vi "IMAQdx Acquisition Template (Host)forRT.vi"() -> ()   [LabVIEW 2016]
uses:
  <vilib>/rvi/interface/nirviOpenFPGA/nirviOpenFPGA.xnode
  <vilib>/rvi/interface/nirviCloseFPGA/nirviCloseFPGA.xnode
  <vilib>/rvi/interface/nirviMethod/nirviMethod.xnode
  <vilib>/FPGAPlugInAG/Dynamic/niLvFpga_Close_Dynamic.vi
  <vilib>/vision/driver/NI_Vision_Acquisition_Software.lvlib
  <resource>/objmgr/imaqdx.rc
  <vilib>/vision/driver/IMAQdx.llb/IMAQdx Acquisition Mode.ctl
  <vilib>/vision/driver/IMAQdx.llb/IMAQdx Buffer Number Mode.ctl
  <vilib>/visionFPGA/NI_VDM_FPGA_Basics.lvlib
  <vilib>/FPGAPlugInAG/Dynamic/niLvFpga_Download_Dynamic.vi
  <vilib>/FPGAPlugInAG/Dynamic/niLvFpga_Run_Dynamic.vi
  <vilib>/rvi/interface/nirviReadWriteControl/nirviReadWriteControl.xnode
  <vilib>/rvi/interface/Simulation/niFpgaSimulationCallBeginRW.vi
  <vilib>/rvi/errors/niLvFpgaAdjustHostInterfaceError.vi
  <vilib>/rvi/errors/niLvFpgaMergeErrorWithErrorCode.vi
  <vilib>/FPGAPlugInAG/Dynamic/niLvFpga_ReadFifo_Dynamic.vi
  <vilib>/FPGAPlugInAG/Dynamic/niLvFpga_ConfigureFifo_Dynamic.vi
  <vilib>/FPGAPlugInAG/Dynamic/niLvFpga_StartFifo_Dynamic.vi
  <vilib>/visionFPGA/Basics/Image Transfer to Target/IMAQ FPGA Image Transfer to Target U32.vi
  <vilib>/visionFPGA/Basics/Configure Image Transfer to Target/IMAQ FPGA Configure Image Transfer to Target U32.vi
  <vilib>/userdefined/High Color/IMAQdx.ctl
  FPGA Bitfiles/ImageProcessingw_FPGATarget2_ImageProcessingw_ZcF2hsHpmf8.lvbitx
  <vilib>/FPGAPlugInAG/roboRIO/niLvFpga_Open_roboRIO.vi
  <vilib>/rvi/interface/common/dynamic/niFpgaDynamicAddResources.vi
panel:
  out "error out":errorcluster
  out "dePixelCount":u32
  out "AllPixelCount":u32
  out "OriImage Err out":errorcluster
  out "Image":T1(plugin-control)
  out "error out 2":errorcluster
  out "Error Out":errorcluster
  in  "Stop":bool
  # "Overview: Demonstrates how to acquire an image from a camera using the IMAQdx API, transfer the image to a FPGA target for processing, and retrieve the processed image for display or further processing on the host.\nRequirements:\n- LabVIEW FPGA\n- Vision Acquisition Software\n- Vision Development Module\nInstructions:\n1. Select a Camera\n2. Run the VI."
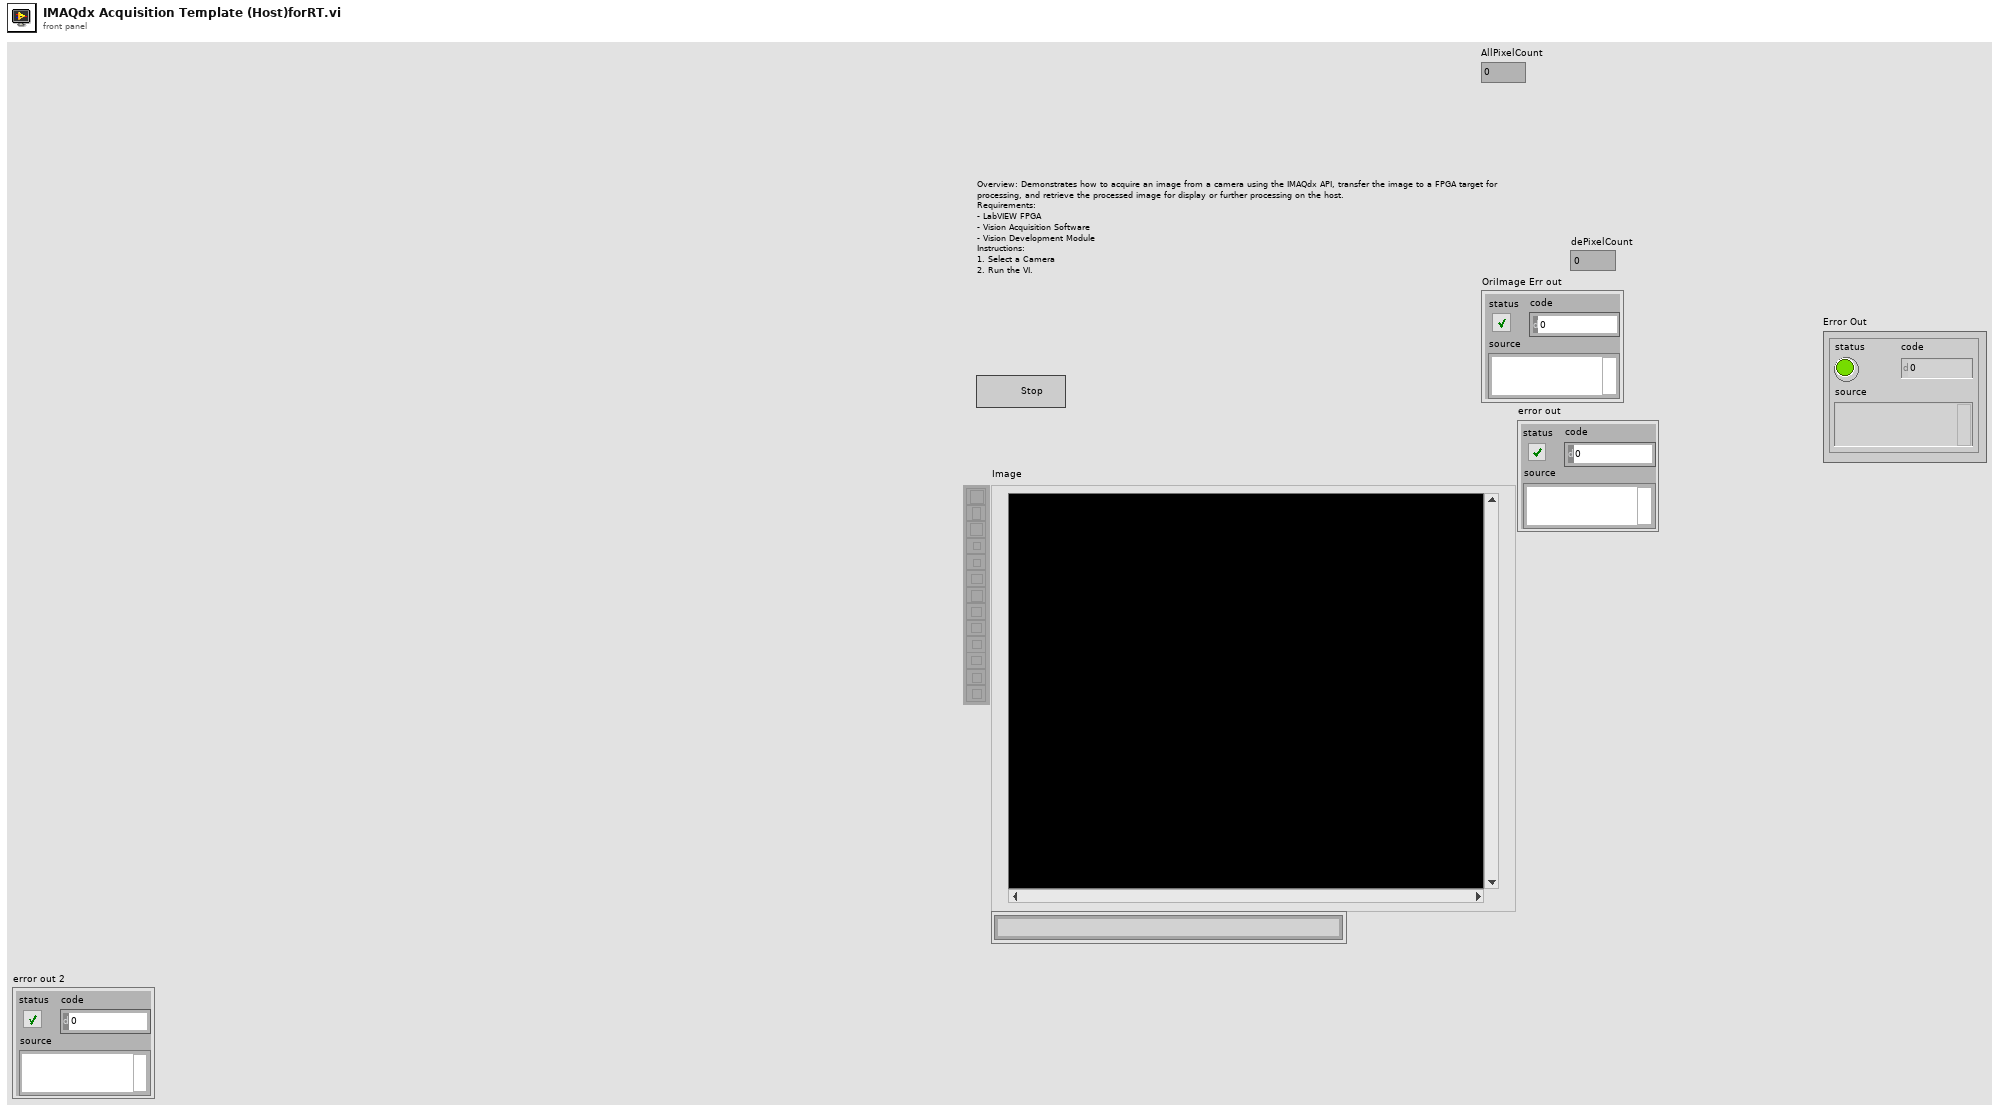
[diagram p1: front panel]
types:
  T1 = typedef "IMAQ Image.ctl" = refnum<image>
  T2 = typedef "IMAQdx.ctl" = refnum<k21>
  T3 = typedef "Image Type" = u32
  T4 = typedef "NI_Vision_Acquisition_Software.lvlib/IMAQdx Acquisition Mode.ctl" = enum32{"One Shot", "Continuous"}
  T5 = typedef "NI_Vision_Acquisition_Software.lvlib/IMAQdx Buffer Number Mode.ctl" = enum32{"Next", "Last", "Buffer Number", "Every", "Last New"}
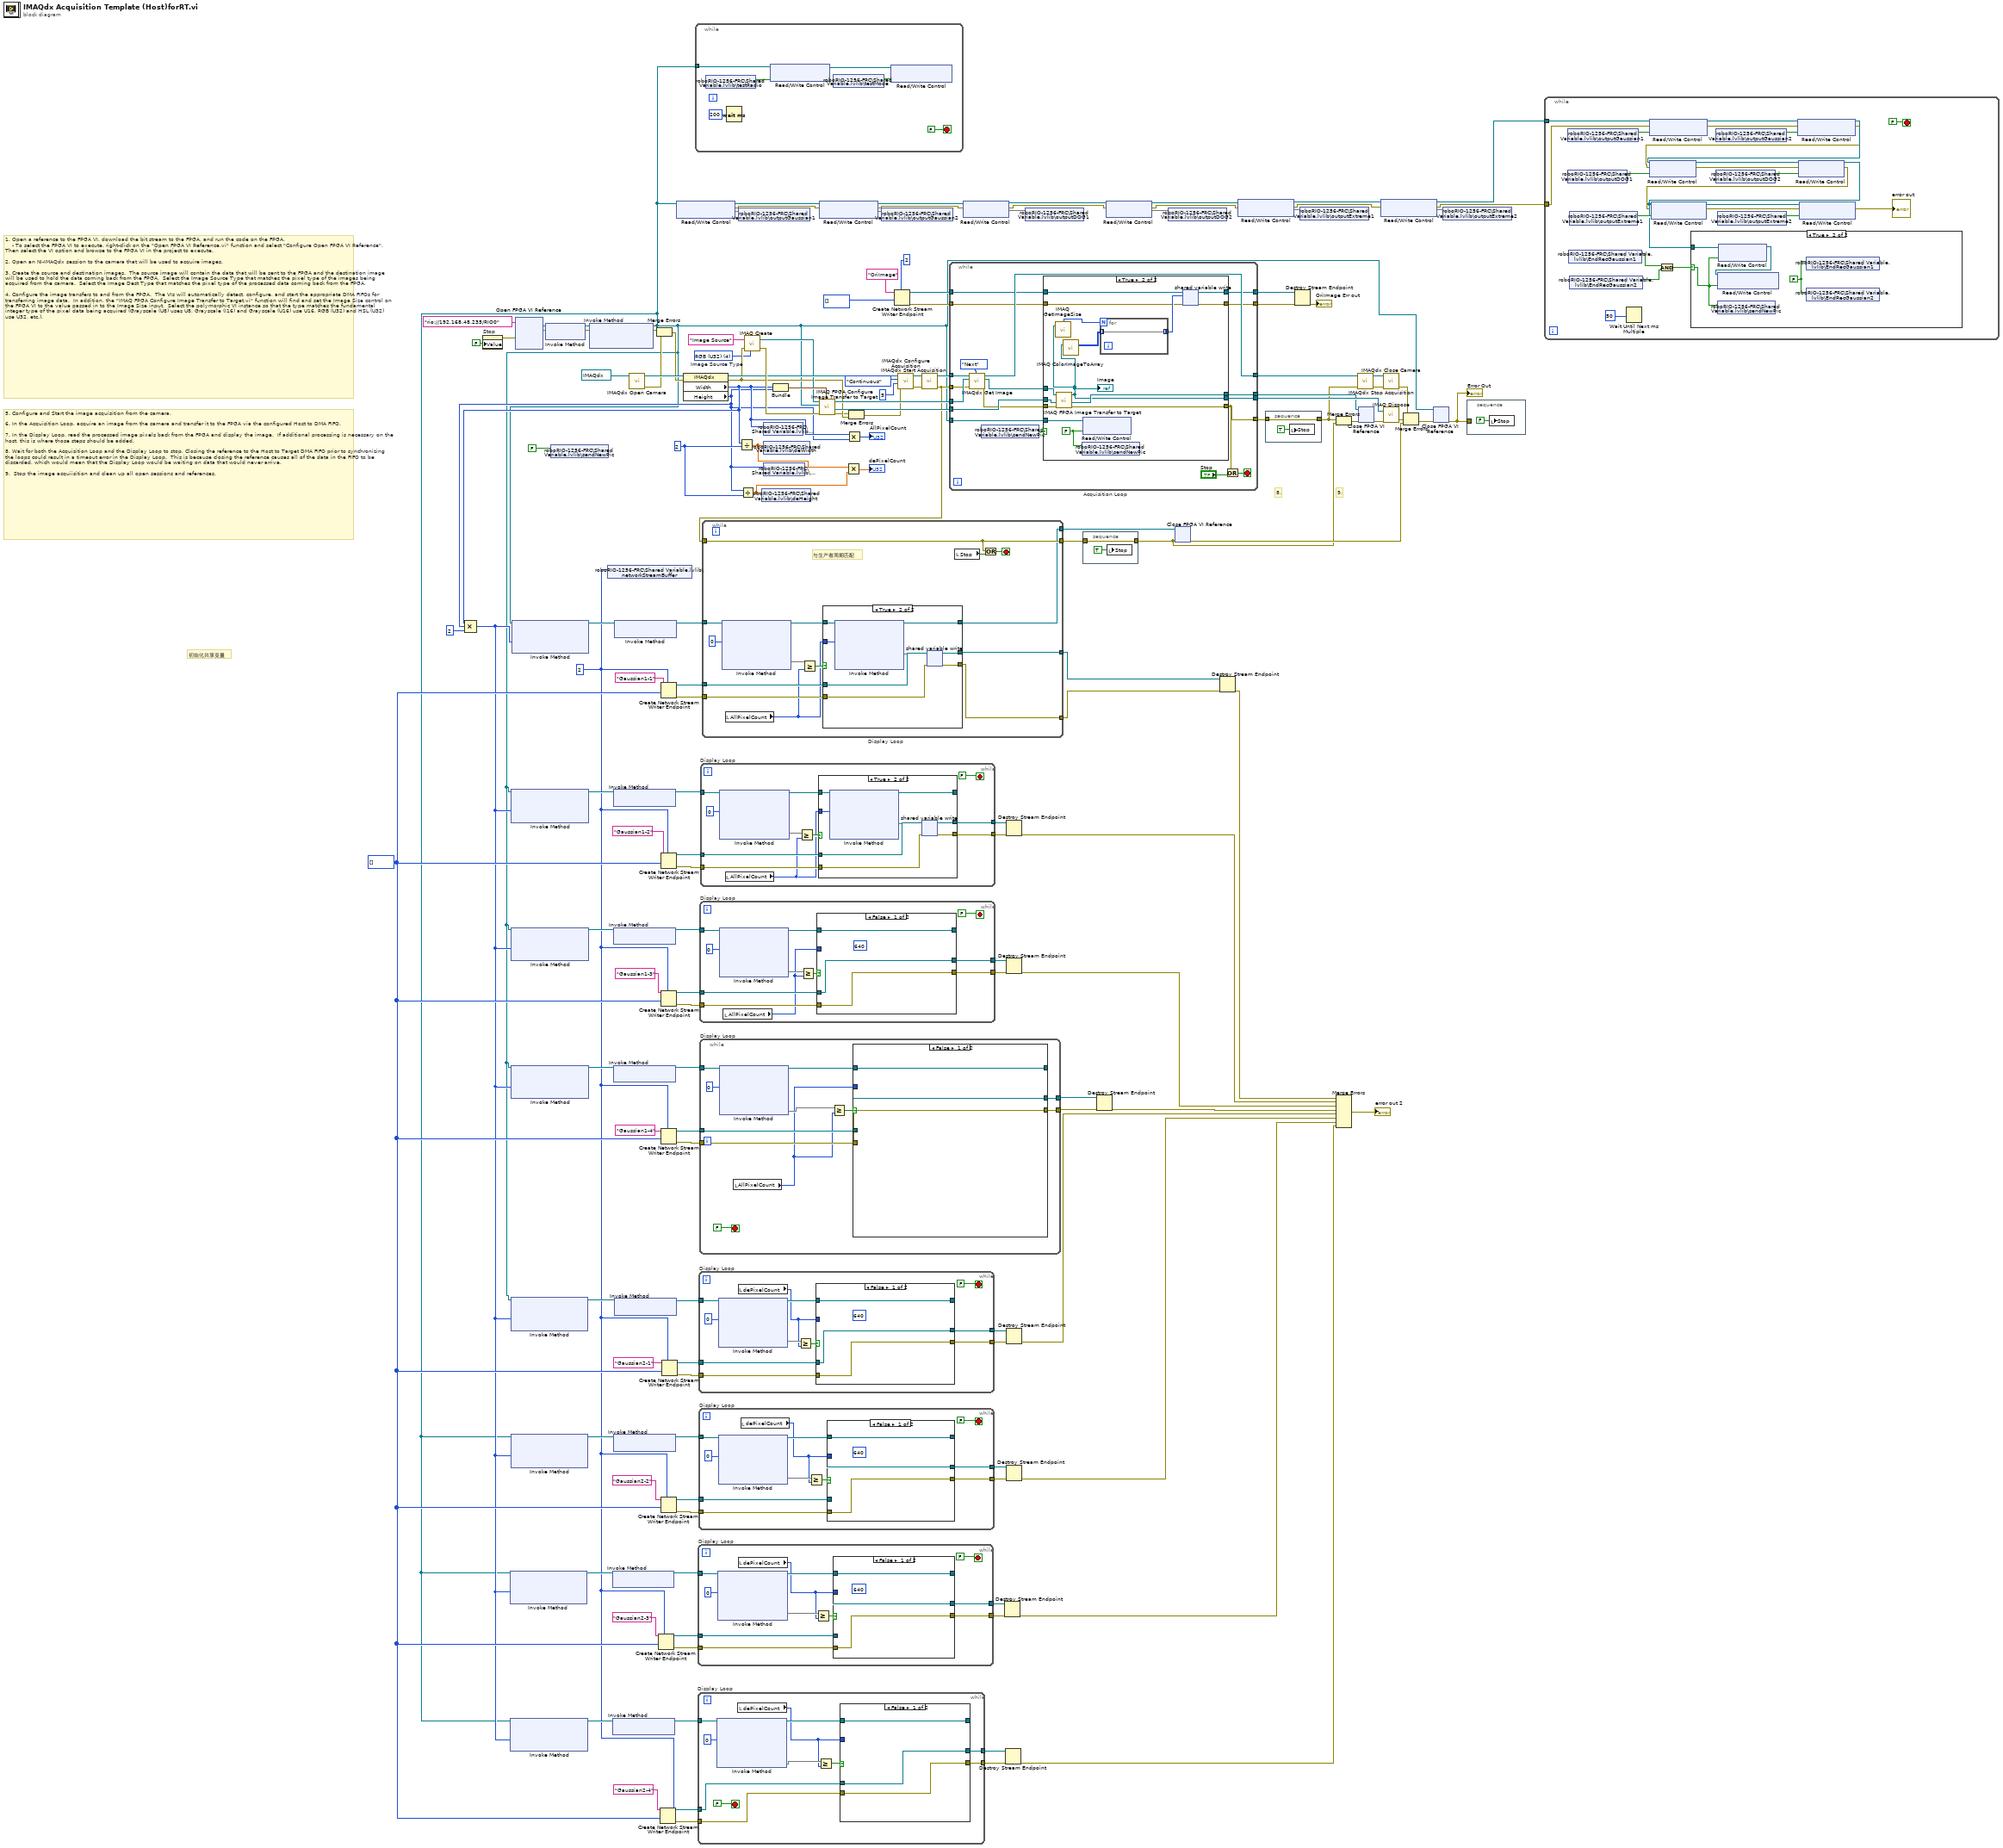
[diagram p0: block diagram]
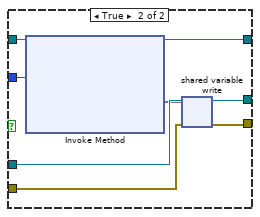
[diagram p3: hidden frame]
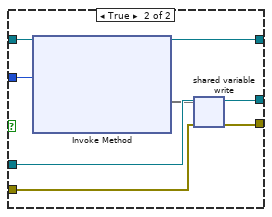
[diagram p4: hidden frame]
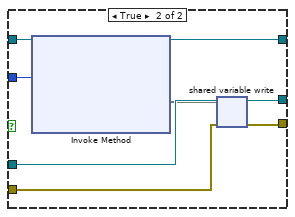
[diagram p5: hidden frame]
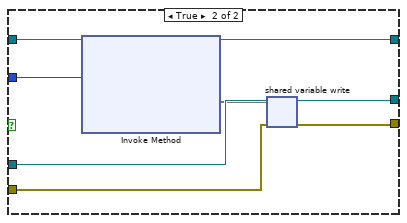
[diagram p6: hidden frame]
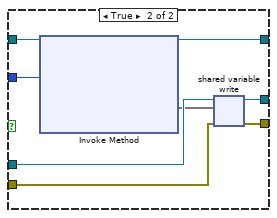
[diagram p7: hidden frame]
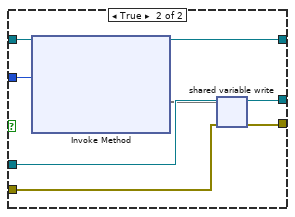
[diagram p8: hidden frame]
diagram:
  w27 = u32 2 ("y")
  w37 = i32[] []
  w34 = 2 ("writer buffer size")
  w114 = T3 4 items=["Grayscale (U8)", "Grayscale (I16)", "Grayscale (SGL)", "Complex (CSG)", "RGB (U32)", "HSL (U32)", "RGB (U64)", "Grayscale (U16)"]  # Image Source Type
  # "初始化共享变量"
  # "5. Configure and Start the image acquisition from the camera.\n\n6. In the Acquisition Loop, acquire an image from the camera and transfer it to the FPGA via the configured Host to DMA FIFO.\n\n7. In the Display Loop, read the processed image pixels back from the FPGA and display the image.  If additional processing is necessary on the host, this is where those steps should be added.\n\n8. Wait for both the Acquisition Loop and the Display Loop to stop. Closing the reference to the Host to Target DMA FIFO prior to synchronizing the loops could result in a timeout error in the Display Loop.  This is because closing the reference causes all of the data in the FIFO to be discarded, which would mean that the Display Loop would be waiting on data that would never arrive.\n\n9.  Stop the image acquiisition and clean up all open sessions and references."
  # "1. Open a reference to the FPGA VI, download the bit stream to the FPGA, and run the code on the FPGA.\n    - To select the FPGA VI to execute, right-click on the \"Open FPGA VI Reference.vi\" function and select \"Configure Open FPGA VI Reference\".  Then select the VI option and browse to the FPGA VI in the project to execute.\n\n2. Open an NI-IMAQdx session to the camera that will be used to acquire images.\n\n3. Create the source and destination images.  The source image will contain the data that will be sent to the FPGA and the destination image will be used to hold the data coming back from the FPGA.  Select the Image Source Type that matches the pixel type of the images being acquired from the camera.  Select the Image Dest Type that matches the pixel type of the processed data coming back from the FPGA.\n\n4. Configure the image transfers to and from the FPGA.  The VIs will automatically detect, configure, and start the appropriate DMA FIFOs for transferring image data.  In addition, the \"IMAQ FPGA Configure Image Transfer to Target.vi\" function will find and set the Image Size control on the FPGA VI to the value passed in to the Image Size input.  Select the polymorphic VI instance so that the type matches the fundamental integer type of the pixel data being acquired (Grayscale (U8) uses U8, Grayscale (I16) and Grayscale (U16) use U16, RGB (U32) and HSL (U32) use U32, etc.)."
  # "9."
  # "8."
  n1 = property on="Stop" class="Bool (strict)"("Value"=FALSE ("Stop")) -> (error out=w149:errorcluster)  [unwired: 2 in, 1 out]
  n2 = xnode "Open FPGA VI Reference"("error in"=w149, "resource name"=tag "rio://192.168.48.235/RIO0") -> ("FPGA VI Reference Out"=w145:refnum<k20>, "error out"=w146:errorcluster)
  n3 = xnode "Invoke Method"("FPGA VI Reference In"=w145, "error in"=w146) -> ("FPGA VI Reference Out"=w148:refnum<k20>, "error out"=w147:errorcluster)
  n4 = shared-variable "roboRIO-1256-FRC\\Shared Variable.lvlib\\sendNewPic"(FALSE) -> ()  [unwired: 1 in, 1 out]
  n5 = xnode "Invoke Method"("FPGA VI Reference In"=w148, "error in"=w147) -> ("FPGA VI Reference Out"=w1:refnum<k20>, "error out"=w134:errorcluster)  [unwired: 1 in]
  n6 = shared-variable "roboRIO-1256-FRC\\Shared Variable.lvlib\\networkStreamBuffer"(w34) -> ()  [unwired: 1 in, 1 out]
  n7 = call <vilib>:"IMAQdx Open Camera.vi"("Session In"=T2 "cam0" ("Camera")) -> ("error out"=w119:errorcluster, "Session Out"=w120:T2)  [unwired: 9 in]
  n8 = Merge Errors(w134, w119) -> (w118:errorcluster)
  n9 = Create Network Stream Writer Endpoint(7:w34, 9:w37, 11:"Gaussian2-3" ("writer name")) -> (0:w41:errorcluster, 3:w40:refnum<k21>)  [unwired: 4 in]
  n10 = Create Network Stream Writer Endpoint(7:w34, 9:w37, 11:"Gaussian2-4" ("writer name")) -> (0:w66:errorcluster, 3:w67:refnum<k21>)  [unwired: 4 in]
  n11 = Create Network Stream Writer Endpoint(7:w34, 9:w37, 11:"Gaussian2-2" ("writer name")) -> (0:w48:errorcluster, 3:w49:refnum<k21>)  [unwired: 4 in]
  n12 = Create Network Stream Writer Endpoint(7:w34, 9:w37, 11:"Gaussian1-1" ("writer name")) -> (0:w98:errorcluster, 3:w97:refnum<k21>)  [unwired: 4 in]
  n13 = Create Network Stream Writer Endpoint(7:w34, 9:w37, 11:"Gaussian1-2" ("writer name")) -> (0:w81:errorcluster, 3:w82:refnum<k21>)  [unwired: 4 in]
  n14 = Create Network Stream Writer Endpoint(7:w34, 9:w37, 11:"Gaussian1-3" ("writer name")) -> (0:w76:errorcluster, 3:w75:refnum<k21>)  [unwired: 4 in]
  n15 = Create Network Stream Writer Endpoint(7:w34, 9:w37, 11:"Gaussian1-4" ("writer name")) -> (0:w60:errorcluster, 3:w61:refnum<k21>)  [unwired: 4 in]
  n16 = Create Network Stream Writer Endpoint(7:w34, 9:w37, 11:"Gaussian2-1" ("writer name")) -> (0:w55:errorcluster, 3:w54:refnum<k21>)  [unwired: 4 in]
  n17 = xnode "Read/Write Control"("FPGA VI Reference In"=w1) -> ("FPGA VI Reference Out"=w24:refnum<k20>, "error out"=w8:errorcluster, "outputGaussian1"=w26)  [unwired: 1 in]
  n18 = property class="IMAQdx"(reference=w120, error in=w118) -> (reference out=w127:T2, error out=w115:errorcluster, "Width"=w14:u32, "Height"=w13:u32)
  n19 = Compound Arithmetic op=MULTIPLY(w14, w13, u32 2 ("value")) -> (w33:u32)
  n20 = xnode "Invoke Method"("FPGA VI Reference In"=w1, "Requested Depth"=w33) -> ("FPGA VI Reference Out"=w42:refnum<k20>)  [unwired: 1 in, 2 out]
  n21 = xnode "Invoke Method"("FPGA VI Reference In"=w1, "Requested Depth"=w33) -> ("FPGA VI Reference Out"=w65:refnum<k20>)  [unwired: 1 in, 2 out]
  n22 = xnode "Invoke Method"("FPGA VI Reference In"=w1, "Requested Depth"=w33) -> ("FPGA VI Reference Out"=w36:refnum<k20>)  [unwired: 1 in, 2 out]
  n23 = xnode "Invoke Method"("FPGA VI Reference In"=w1, "Requested Depth"=w33) -> ("FPGA VI Reference Out"=w47:refnum<k20>)  [unwired: 1 in, 2 out]
  n24 = xnode "Invoke Method"("FPGA VI Reference In"=w1, "Requested Depth"=w33) -> ("FPGA VI Reference Out"=w80:refnum<k20>)  [unwired: 1 in, 2 out]
  n25 = xnode "Invoke Method"("FPGA VI Reference In"=w1, "Requested Depth"=w33) -> ("FPGA VI Reference Out"=w77:refnum<k20>)  [unwired: 1 in, 2 out]
  n26 = xnode "Invoke Method"("FPGA VI Reference In"=w1, "Requested Depth"=w33) -> ("FPGA VI Reference Out"=w59:refnum<k20>)  [unwired: 1 in, 2 out]
  n27 = xnode "Invoke Method"("FPGA VI Reference In"=w1, "Requested Depth"=w33) -> ("FPGA VI Reference Out"=w104:refnum<k20>)  [unwired: 1 in, 2 out]
  n28 = xnode "Invoke Method"("FPGA VI Reference In"=w42) -> ("FPGA VI Reference Out"=w43:refnum<k20>)  [unwired: 1 in, 1 out]
  n29 = xnode "Invoke Method"("FPGA VI Reference In"=w65) -> ("FPGA VI Reference Out"=w64:refnum<k20>)  [unwired: 1 in, 1 out]
  n30 = xnode "Invoke Method"("FPGA VI Reference In"=w47) -> ("FPGA VI Reference Out"=w46:refnum<k20>)  [unwired: 1 in, 1 out]
  n31 = xnode "Invoke Method"("FPGA VI Reference In"=w80) -> ("FPGA VI Reference Out"=w79:refnum<k20>)  [unwired: 1 in, 1 out]
  n32 = xnode "Invoke Method"("FPGA VI Reference In"=w77) -> ("FPGA VI Reference Out"=w78:refnum<k20>)  [unwired: 1 in, 1 out]
  n33 = xnode "Invoke Method"("FPGA VI Reference In"=w59) -> ("FPGA VI Reference Out"=w58:refnum<k20>)  [unwired: 1 in, 1 out]
  n34 = xnode "Invoke Method"("FPGA VI Reference In"=w104) -> ("FPGA VI Reference Out"=w103:refnum<k20>)  [unwired: 1 in, 1 out]
  n35 = xnode "Invoke Method"("FPGA VI Reference In"=w36) -> ("FPGA VI Reference Out"=w35:refnum<k20>)  [unwired: 1 in, 1 out]
  n36 = while {
    tunnel: w1 -> [w151]
    stop <- FALSE stop-if-true
    n37 = shared-variable "roboRIO-1256-FRC\\Shared Variable.lvlib\\testRadio"() -> (w152:bool)  [unwired: 1 in, 1 out]
    n38 = Wait (ms)(milliseconds to wait=u32 200) -> ()  [unwired: 1 out]
    n39 = xnode "Read/Write Control"("FPGA VI Reference In"=w151, "Radio LED Status"=w152) -> ("FPGA VI Reference Out"=w156:refnum<k20>)  [unwired: 1 in, 1 out]
    n40 = shared-variable "roboRIO-1256-FRC\\Shared Variable.lvlib\\testMode"() -> (w153:bool)  [unwired: 1 in, 1 out]
    n41 = xnode "Read/Write Control"("FPGA VI Reference In"=w156, "Comm LED Status"=w153) -> ()  [unwired: 1 in, 2 out]
  }
  n42 = while "Display Loop" {
    tunnel: [w167] -> w70
    tunnel: w66 -> [w166]
    tunnel: w67 -> [w165]
    tunnel: [w161] -> w69
    tunnel: w64 -> [w160]
    stop <- FALSE stop-if-true
    n43 = xnode "Invoke Method"("FPGA VI Reference In"=w160, "Number of Elements"=u32 0) -> ("FPGA VI Reference Out"=w163:refnum<k20>, "Elements Remaining"=w158)  [unwired: 2 in, 2 out]
    n44 = local read "dePixelCount"() -> (w157:u32)
    n45 = Greater Or Equal?(x=w158, y=w157) -> (x >= y?=w159:bool)
    n46 = case shown="False" w159 {
      tunnel: w163 -> [w168 w178]
      tunnel: [w170 w177] -> w167
      tunnel: w166 -> [w169 w176]
      tunnel: w165 -> [w170 w175]
      tunnel: [w169 w174] -> w161
      tunnel: [w168 w173] -> _
      tunnel: w157 -> [_ w171]
      frame False {
      }
      frame True {
        n47 = xnode "Invoke Method"("FPGA VI Reference In"=w178, "Number of Elements"=w171) -> ("FPGA VI Reference Out"=w173:refnum<k20>, "Data"=w172:void[])  [unwired: 2 in, 2 out]
        n48 = shared-variable-write(w175, w176, w172) -> (w177:refnum<k21>, w174:errorcluster)  [unwired: 1 in, 1 out]
      }
    }
  }
  n49 = while "Display Loop" {
    tunnel: [w189] -> w38
    tunnel: w41 -> [w188]
    tunnel: w40 -> [w187]
    tunnel: [w183] -> w39
    tunnel: w43 -> [w182]
    stop <- FALSE stop-if-true
    (unwired) u32 640 ("Number of Elements")
    n50 = xnode "Invoke Method"("FPGA VI Reference In"=w182, "Number of Elements"=u32 0) -> ("FPGA VI Reference Out"=w185:refnum<k20>, "Elements Remaining"=w180)  [unwired: 2 in, 2 out]
    n51 = local read "dePixelCount"() -> (w179:u32)
    n52 = Greater Or Equal?(x=w180, y=w179) -> (x >= y?=w181:bool)
    n53 = case shown="False" w181 {
      tunnel: w185 -> [w190 w200]
      tunnel: [w192 w199] -> w189
      tunnel: w188 -> [w191 w198]
      tunnel: w187 -> [w192 w197]
      tunnel: [w191 w196] -> w183
      tunnel: [w190 w194] -> _
      tunnel: w179 -> [_ w193]
      frame False {
      }
      frame True {
        n54 = xnode "Invoke Method"("FPGA VI Reference In"=w200, "Number of Elements"=w193) -> ("FPGA VI Reference Out"=w194:refnum<k20>, "Data"=w195:void[])  [unwired: 2 in, 2 out]
        n55 = shared-variable-write(w197, w198, w195) -> (w199:refnum<k21>, w196:errorcluster)  [unwired: 1 in, 1 out]
      }
    }
  }
  n56 = while "Display Loop" {
    tunnel: [w211] -> w52
    tunnel: w55 -> [w210]
    tunnel: w54 -> [w209]
    tunnel: [w205] -> w53
    tunnel: w35 -> [w204]
    stop <- FALSE stop-if-true
    (unwired) u32 640 ("Number of Elements")
    n57 = xnode "Invoke Method"("FPGA VI Reference In"=w204, "Number of Elements"=u32 0) -> ("FPGA VI Reference Out"=w207:refnum<k20>, "Elements Remaining"=w202)  [unwired: 2 in, 2 out]
    n58 = local read "dePixelCount"() -> (w201:u32)
    n59 = Greater Or Equal?(x=w202, y=w201) -> (x >= y?=w203:bool)
    n60 = case shown="False" w203 {
      tunnel: w207 -> [w212 w222]
      tunnel: [w214 w221] -> w211
      tunnel: w210 -> [w213 w220]
      tunnel: w209 -> [w214 w219]
      tunnel: [w213 w218] -> w205
      tunnel: [w212 w216] -> _
      tunnel: w201 -> [_ w215]
      frame False {
      }
      frame True {
        n61 = xnode "Invoke Method"("FPGA VI Reference In"=w222, "Number of Elements"=w215) -> ("FPGA VI Reference Out"=w216:refnum<k20>, "Data"=w217:void[])  [unwired: 2 in, 2 out]
        n62 = shared-variable-write(w219, w220, w217) -> (w221:refnum<k21>, w218:errorcluster)  [unwired: 1 in, 1 out]
      }
    }
  }
  n63 = while "Display Loop" {
    tunnel: [w233] -> w51
    tunnel: w48 -> [w232]
    tunnel: w49 -> [w231]
    tunnel: [w227] -> w50
    tunnel: w46 -> [w226]
    stop <- FALSE stop-if-true
    (unwired) u32 640 ("Number of Elements")
    n64 = xnode "Invoke Method"("FPGA VI Reference In"=w226, "Number of Elements"=u32 0) -> ("FPGA VI Reference Out"=w229:refnum<k20>, "Elements Remaining"=w224)  [unwired: 2 in, 2 out]
    n65 = local read "dePixelCount"() -> (w223:u32)
    n66 = Greater Or Equal?(x=w224, y=w223) -> (x >= y?=w225:bool)
    n67 = case shown="False" w225 {
      tunnel: w229 -> [w234 w244]
      tunnel: [w236 w243] -> w233
      tunnel: w232 -> [w235 w242]
      tunnel: w231 -> [w236 w241]
      tunnel: [w235 w240] -> w227
      tunnel: [w234 w238] -> _
      tunnel: w223 -> [_ w237]
      frame False {
      }
      frame True {
        n68 = xnode "Invoke Method"("FPGA VI Reference In"=w244, "Number of Elements"=w237) -> ("FPGA VI Reference Out"=w238:refnum<k20>, "Data"=w239:void[])  [unwired: 2 in, 2 out]
        n69 = shared-variable-write(w241, w242, w239) -> (w243:refnum<k21>, w240:errorcluster)  [unwired: 1 in, 1 out]
      }
    }
  }
  n70 = while "Display Loop" {
    tunnel: [w255] -> w72
    tunnel: w76 -> [w254]
    tunnel: w75 -> [w253]
    tunnel: [w249] -> w73
    tunnel: w78 -> [w248]
    stop <- FALSE stop-if-true
    (unwired) u32 640 ("Number of Elements")
    n71 = xnode "Invoke Method"("FPGA VI Reference In"=w248, "Number of Elements"=u32 0) -> ("FPGA VI Reference Out"=w251:refnum<k20>, "Elements Remaining"=w246)  [unwired: 2 in, 2 out]
    n72 = local read "AllPixelCount"() -> (w245:u32)
    n73 = Greater Or Equal?(x=w246, y=w245) -> (x >= y?=w247:bool)
    n74 = case shown="False" w247 {
      tunnel: w251 -> [w256 w266]
      tunnel: [w258 w265] -> w255
      tunnel: w254 -> [w257 w264]
      tunnel: w253 -> [w258 w263]
      tunnel: [w257 w262] -> w249
      tunnel: [w256 w260] -> _
      tunnel: w245 -> [_ w259]
      frame False {
      }
      frame True {
        n75 = xnode "Invoke Method"("FPGA VI Reference In"=w266, "Number of Elements"=w259) -> ("FPGA VI Reference Out"=w260:refnum<k20>, "Data"=w261:void[])  [unwired: 2 in, 2 out]
        n76 = shared-variable-write(w263, w264, w261) -> (w265:refnum<k21>, w262:errorcluster)  [unwired: 1 in, 1 out]
      }
    }
  }
  n77 = while "Display Loop" {
    tunnel: [w277] -> w63
    tunnel: w60 -> [w276]
    tunnel: w61 -> [w275]
    tunnel: [w271] -> w62
    tunnel: w58 -> [w270]
    stop <- FALSE stop-if-true
    n78 = xnode "Invoke Method"("FPGA VI Reference In"=w270, "Number of Elements"=u32 0) -> ("FPGA VI Reference Out"=w273:refnum<k20>, "Elements Remaining"=w268)  [unwired: 2 in, 2 out]
    n79 = local read "AllPixelCount"() -> (w267:u32)
    n80 = Greater Or Equal?(x=w268, y=w267) -> (x >= y?=w269:bool)
    n81 = case shown="False" w269 {
      tunnel: w273 -> [w278 w282]
      tunnel: [w280 w288] -> w277
      tunnel: w276 -> [w279 w287]
      tunnel: w275 -> [w280 w286]
      tunnel: [w279 w285] -> w271
      tunnel: [w278 w284] -> _
      tunnel: w267 -> [_ w281]
      frame False {
      }
      frame True {
        n82 = xnode "Invoke Method"("FPGA VI Reference In"=w282, "Number of Elements"=w281) -> ("FPGA VI Reference Out"=w284:refnum<k20>, "Data"=w283:void[])  [unwired: 2 in, 2 out]
        n83 = shared-variable-write(w286, w287, w283) -> (w288:refnum<k21>, w285:errorcluster)  [unwired: 1 in, 1 out]
      }
    }
  }
  n84 = while "Display Loop" {
    tunnel: [w299] -> w88
    tunnel: w81 -> [w298]
    tunnel: w82 -> [w297]
    tunnel: [w293] -> w87
    tunnel: w79 -> [w292]
    stop <- FALSE stop-if-true
    (unwired) u32 640 ("Number of Elements")
    n85 = xnode "Invoke Method"("FPGA VI Reference In"=w292, "Number of Elements"=u32 0) -> ("FPGA VI Reference Out"=w295:refnum<k20>, "Elements Remaining"=w290)  [unwired: 2 in, 2 out]
    n86 = local read "AllPixelCount"() -> (w289:u32)
    n87 = Greater Or Equal?(x=w290, y=w289) -> (x >= y?=w291:bool)
    n88 = case shown="True" w291 {
      tunnel: w295 -> [w300 w310]
      tunnel: [w302 w309] -> w299
      tunnel: w298 -> [w301 w308]
      tunnel: w297 -> [w302 w307]
      tunnel: [w301 w306] -> w293
      tunnel: [w300 w304] -> _
      tunnel: w289 -> [_ w303]
      frame False {
      }
      frame True {
        n89 = xnode "Invoke Method"("FPGA VI Reference In"=w310, "Number of Elements"=w303) -> ("FPGA VI Reference Out"=w304:refnum<k20>, "Data"=w305:void[])  [unwired: 2 in, 2 out]
        n90 = shared-variable-write(w307, w308, w305) -> (w309:refnum<k21>, w306:errorcluster)  [unwired: 1 in, 1 out]
      }
    }
  }
  n91 = shared-variable "roboRIO-1256-FRC\\Shared Variable.lvlib\\outputGaussian1"(w26) -> ()  [unwired: 1 in, 1 out]
  n92 = Divide(x=w14, y=w27) -> (x/y=w10:dbl)
  n93 = Divide(x=w13, y=w27) -> (x/y=w9:dbl)
  n94 = call "IMAQ Create"("Image Name"="Image Source", "Image Type"=w114, "error in (no error)"=w115) -> ("New Image"=w125:T1, "error out"=w133:errorcluster)  [unwired: 2 in]
  n95 = shared-variable "roboRIO-1256-FRC\\Shared Variable.lvlib\\deHeight"(w9) -> ()  [unwired: 1 in, 1 out]
  n96 = shared-variable "roboRIO-1256-FRC\\Shared Variable.lvlib\\Width"(w14) -> ()  [unwired: 1 in, 1 out]
  n97 = shared-variable "roboRIO-1256-FRC\\Shared Variable.lvlib\\deWidth"(w10) -> ()  [unwired: 1 in, 1 out]
  n98 = shared-variable "roboRIO-1256-FRC\\Shared Variable.lvlib\\Height"(w13) -> ()  [unwired: 1 in, 1 out]
  n99 = Bundle("Width"=w14, "Height"=w13) -> (w132:cluster{"Width":u32, "Height":u32})  [unwired: 1 in]
  n100 = xnode "Read/Write Control"("FPGA VI Reference In"=w24, "error in"=w8) -> ("FPGA VI Reference Out"=w20:refnum<k20>, "error out"=w7:errorcluster, "outputGaussian2"=w25)
  n101 = call-poly <vilib>:"IMAQ FPGA Configure Image Transfer to Target.vi"("Image Size"=w132, "error in (no error)"=w133, "FPGA VI Reference In"=w1, "Image"=w125) -> ("error out"=w108:errorcluster, "DMA FIFO Reference Out"=w143:refnum<k20>, "Image Out"=w144:T1)  [unwired: 4 in, 1 out]
  n102 = Multiply(x=w10, y=w9) -> (x*y=→"dePixelCount":dbl)
  n103 = Multiply(x=w14, y=w13) -> (x*y=→"AllPixelCount":u32)
  n104 = Merge Errors(w108, w115) -> (w107:errorcluster)
  n105 = shared-variable "roboRIO-1256-FRC\\Shared Variable.lvlib\\outputGaussian2"(w25) -> ()  [unwired: 1 in, 1 out]
  n106 = Create Network Stream Writer Endpoint(7:2 ("writer buffer size"), 9:i32[] [], 11:"OriImage" ("writer name")) -> (0:w92:errorcluster, 3:w93:refnum<k21>)  [unwired: 4 in]
  n107 = call <vilib>:"IMAQdx Configure Acquisition.vi"("error in"=w107, "Number of Buffers"=u32 5, "Continuous?"=IMAQdx_Acquisition_Mode."Continuous", "Session In"=w127) -> ("error out"=w130:errorcluster, "Session Out"=w131:T2)  [unwired: 6 in]
  n108 = call <vilib>:"IMAQdx Start Acquisition.vi"("error in"=w130, "Session In"=w131) -> ("error out"=w106:errorcluster, "Session Out"=w126:T2)  [unwired: 8 in]
  n109 = while "Display Loop" {
    tunnel: w106 -> [w323]
    tunnel: [w315] -> w140
    tunnel: [w323] -> w139
    tunnel: w103 -> [w316]
    tunnel: [w318] -> w100
    tunnel: [w321] -> w99
    tunnel: w98 -> [w320]
    tunnel: w97 -> [w319]
    stop <- w324 stop-if-true
    (unwired) u32 640 ("Number of Elements")
    # "与生产者周期匹配"
    n110 = xnode "Invoke Method"("FPGA VI Reference In"=w316, "Number of Elements"=u32 0) -> ("FPGA VI Reference Out"=w314:refnum<k20>, "Elements Remaining"=w311)  [unwired: 2 in, 2 out]
    n111 = local read "AllPixelCount"() -> (w312:u32)
    n112 = Greater Or Equal?(x=w311, y=w312) -> (x >= y?=w313:bool)
    n113 = case shown="True" w313 {
      tunnel: w314 -> [w325 w335]
      tunnel: [w327 w334] -> w321
      tunnel: w320 -> [w326 w333]
      tunnel: w319 -> [w327 w332]
      tunnel: [w326 w331] -> w318
      tunnel: [w325 w329] -> w315
      tunnel: w312 -> [_ w328]
      frame False {
      }
      frame True {
        n114 = xnode "Invoke Method"("FPGA VI Reference In"=w335, "Number of Elements"=w328) -> ("FPGA VI Reference Out"=w329:refnum<k20>, "Data"=w330:void[])  [unwired: 2 in, 2 out]
        n115 = shared-variable-write(w332, w333, w330) -> (w334:refnum<k21>, w331:errorcluster)  [unwired: 1 in, 1 out]
      }
    }
    n116 = local read "Stop"() -> (w322:bool)
    n117 = Or(x=w323, y=w322) -> (x .or. y?=w324:bool)
  }
  n118 = while "Acquisition Loop" {
    tunnel: [w345] -> w112
    tunnel: w144 -> [w350]
    tunnel: w143 -> [w347]
    tunnel: [w346] -> w113
    tunnel: [w343] -> w142
    tunnel: w126 -> [w351]
    tunnel: [w349] -> w122
    tunnel: w106 -> [w348]
    tunnel: w1 -> [w341]
    tunnel: w93 -> [w340]
    tunnel: w92 -> [w339]
    tunnel: [w338] -> w91
    tunnel: [w337] -> w90
    stop <- w353 stop-if-true
    n119 = call <vilib>:"IMAQdx Get Image.vi"("Buffer Number Mode (Next)"=IMAQdx_Buffer_Number_Mode."Next", "error in"=w348, "Image In"=w350, "Session In"=w351) -> ("error out"=w342:errorcluster, "Image Out"=w344:T1, "Session Out"=w349:T2)  [unwired: 4 in, 1 out]
    n120 = shared-variable "roboRIO-1256-FRC\\Shared Variable.lvlib\\sendNewPic"() -> (w336:bool)  [unwired: 1 in, 1 out]
    n121 = case shown="True" w336 {
      tunnel: w347 -> [w359 w374]
      tunnel: [w359 w370] -> w346
      tunnel: [w358 w371] -> w345
      tunnel: w344 -> [w357 w373]
      tunnel: [w357 w365] -> w343
      tunnel: w342 -> [w358 w372]
      tunnel: w341 -> [_ w368]
      tunnel: w340 -> [w356 w363]
      tunnel: w339 -> [w355 w362]
      tunnel: [w356 w361] -> w338
      tunnel: [w355 w360] -> w337
      frame False {
      }
      frame True {
        w369 = FALSE ("EndOfImage")
        n122 = call-poly <vilib>:"IMAQ FPGA Image Transfer to Target.vi"("error in (no error)"=w372, "DMA FIFO Reference In"=w374, "Image"=w373) -> ("error out"=w371:errorcluster, "DMA FIFO Reference Out"=w370:refnum<k20>, "Image Out"=w365:T1)  [unwired: 6 in]
        "Image" <- w365
        n123 = call "IMAQ GetImageSize"("Image"=w365) -> ("X Resolution"=w367:i32)  [unwired: 3 in, 2 out]
        n124 = call "IMAQ ColorImageToArray"("Image"=w365) -> ("Image Pixels (U32)"=w366:u32[][])  [unwired: 3 in, 2 out]
        n125 = shared-variable "roboRIO-1256-FRC\\Shared Variable.lvlib\\sendNewPic"(w369) -> ()  [unwired: 1 in, 1 out]
        n126 = xnode "Read/Write Control"("FPGA VI Reference In"=w368, "StartOfImage"=w369) -> ()  [unwired: 1 in, 2 out]
        n127 = for {
          N: w367 -> [_]
          tunnel: w366 -> [w375] mode=indexing
          tunnel: [w375] -> w364 mode=concatenating
        }
        n128 = shared-variable-write(w363, w362, w364) -> (w361:refnum<k21>, w360:errorcluster)  [unwired: 1 in, 1 out]
      }
    }
    n129 = Or(x=w345, y="Stop") -> (x .or. y?=w353:bool)
  }
  n130 = xnode "Read/Write Control"("FPGA VI Reference In"=w20, "error in"=w7) -> ("FPGA VI Reference Out"=w23:refnum<k20>, "error out"=w6:errorcluster, "outputDOG1"=w21)
  n131 = Destroy Stream Endpoint(8:w39, 11:w38) -> (0:w29:errorcluster)
  n132 = Destroy Stream Endpoint(8:w69, 11:w70) -> (0:w28:errorcluster)
  n133 = Destroy Stream Endpoint(8:w50, 11:w51) -> (0:w30:errorcluster)
  n134 = Destroy Stream Endpoint(8:w87, 11:w88) -> (0:w84:errorcluster)
  n135 = Destroy Stream Endpoint(8:w73, 11:w72) -> (0:w71:errorcluster)
  n136 = Destroy Stream Endpoint(8:w53, 11:w52) -> (0:w31:errorcluster)
  n137 = shared-variable "roboRIO-1256-FRC\\Shared Variable.lvlib\\outputDOG1"(w21) -> ()  [unwired: 1 in, 1 out]
  n138 = stacked-sequence {
    tunnel: w139 -> [w376]
    tunnel: [w376] -> w111
    frame #0 {
      n139 = local write "Stop"(TRUE ("Stop")) -> ()
    }
  }
  n140 = Destroy Stream Endpoint(8:w62, 11:w63) -> (0:w32:errorcluster)
  n141 = xnode "Read/Write Control"("FPGA VI Reference In"=w23, "error in"=w6) -> ("FPGA VI Reference Out"=w16:refnum<k20>, "error out"=w5:errorcluster, "outputDOG2"=w22)
  n142 = shared-variable "roboRIO-1256-FRC\\Shared Variable.lvlib\\outputDOG2"(w22) -> ()  [unwired: 1 in, 1 out]
  n143 = xnode "Close FPGA VI Reference"("FPGA VI Reference In"=w140, "error in"=w111) -> ("error out"=w138:errorcluster)
  n144 = Destroy Stream Endpoint(8:w100, 11:w99) -> (0:w85:errorcluster)
  n145 = xnode "Read/Write Control"("FPGA VI Reference In"=w16, "error in"=w5) -> ("FPGA VI Reference Out"=w17:refnum<k20>, "error out"=w4:errorcluster, "outputExtreme1"=w19)
  n146 = stacked-sequence {
    tunnel: w112 -> [w378]
    tunnel: [w378] -> w109
    frame #0 {
      n147 = local write "Stop"(TRUE ("Stop")) -> ()
    }
  }
  n148 = Destroy Stream Endpoint(8:w90, 11:w91) -> (0:→"OriImage Err out":errorcluster)
  n149 = shared-variable "roboRIO-1256-FRC\\Shared Variable.lvlib\\outputExtreme1"(w19) -> ()  [unwired: 1 in, 1 out]
  n150 = Merge Errors(w109, w111) -> (w110:errorcluster)
  n151 = Merge Errors(w85, w84, w71, w32, w31, w30, w29, w28) -> (→"error out 2":errorcluster)
  n152 = call <vilib>:"IMAQdx Stop Acquisition.vi"("error in"=w109, "Session In"=w122) -> ("error out"=w123:errorcluster, "Session Out"=w124:T2)  [unwired: 8 in]
  n153 = xnode "Close FPGA VI Reference"("FPGA VI Reference In"=w113, "error in"=w110) -> ("error out"=w141:errorcluster)
  n154 = xnode "Read/Write Control"("FPGA VI Reference In"=w17, "error in"=w4) -> ("FPGA VI Reference Out"=w15:refnum<k20>, "error out"=w3:errorcluster, "outputExtreme2"=w18)
  n155 = call <vilib>:"IMAQdx Close Camera.vi"("error in"=w123, "Session In"=w124) -> ("error out"=w121:errorcluster)  [unwired: 9 in]
  n156 = call "IMAQ Dispose"("Image"=w142, "error in (no error)"=w141) -> ("error out"=w137:errorcluster)  [unwired: 4 in]
  n157 = Merge Errors(w121, w137, w138) -> (w117:errorcluster)
  n158 = xnode "Close FPGA VI Reference"("FPGA VI Reference In"=w1, "error in"=w117) -> ("error out"=w116:errorcluster)
  "Error Out" <- w116
  n159 = shared-variable "roboRIO-1256-FRC\\Shared Variable.lvlib\\outputExtreme2"(w18) -> ()  [unwired: 1 in, 1 out]
  n160 = stacked-sequence {
    tunnel: w116 -> [_]
    frame #0 {
      n161 = local write "Stop"(FALSE ("Stop")) -> ()
    }
  }
  n162 = while {
    tunnel: w15 -> [w403]
    tunnel: w3 -> [w387]
    stop <- FALSE stop-if-true
    n163 = shared-variable "roboRIO-1256-FRC\\Shared Variable.lvlib\\outputGaussian1"() -> (w404:bool)  [unwired: 1 in, 1 out]
    n164 = shared-variable "roboRIO-1256-FRC\\Shared Variable.lvlib\\outputDOG1"() -> (w400:bool)  [unwired: 1 in, 1 out]
    n165 = shared-variable "roboRIO-1256-FRC\\Shared Variable.lvlib\\EndRecGaussian1"() -> (w392:bool)  [unwired: 1 in, 1 out]
    n166 = shared-variable "roboRIO-1256-FRC\\Shared Variable.lvlib\\outputExtreme1"() -> (w394:bool)  [unwired: 1 in, 1 out]
    n167 = shared-variable "roboRIO-1256-FRC\\Shared Variable.lvlib\\EndRecGaussian2"() -> (w391:bool)  [unwired: 1 in, 1 out]
    n168 = Wait Until Next ms Multiple(millisecond multiple=u32 50 ("milliseconds to wait")) -> ()  [unwired: 1 out]
    n169 = xnode "Read/Write Control"("FPGA VI Reference In"=w403, "error in"=w387, "outputGaussian1"=w404) -> ("FPGA VI Reference Out"=w402:refnum<k20>, "error out"=w386:errorcluster)
    n170 = And(x=w392, y=w391) -> (x .and. y?=w390:bool)
    n171 = shared-variable "roboRIO-1256-FRC\\Shared Variable.lvlib\\outputGaussian2"() -> (w401:bool)  [unwired: 1 in, 1 out]
    n172 = shared-variable "roboRIO-1256-FRC\\Shared Variable.lvlib\\outputDOG2"() -> (w398:bool)  [unwired: 1 in, 1 out]
    n173 = shared-variable "roboRIO-1256-FRC\\Shared Variable.lvlib\\outputExtreme2"() -> (w396:bool)  [unwired: 1 in, 1 out]
    n174 = xnode "Read/Write Control"("FPGA VI Reference In"=w402, "error in"=w386, "outputGaussian2"=w401) -> ("FPGA VI Reference Out"=w397:refnum<k20>, "error out"=w385:errorcluster)
    n175 = xnode "Read/Write Control"("FPGA VI Reference In"=w397, "error in"=w385, "outputDOG1"=w400) -> ("FPGA VI Reference Out"=w399:refnum<k20>, "error out"=w384:errorcluster)
    n176 = xnode "Read/Write Control"("FPGA VI Reference In"=w399, "error in"=w384, "outputDOG2"=w398) -> ("FPGA VI Reference Out"=w389:refnum<k20>, "error out"=w383:errorcluster)
    n177 = xnode "Read/Write Control"("FPGA VI Reference In"=w389, "error in"=w383, "outputExtreme1"=w394) -> ("FPGA VI Reference Out"=w395:refnum<k20>, "error out"=w382:errorcluster)
    n178 = case shown="True" w390 {
      selector: w390 -> [_ w407]
      tunnel: w389 -> [_ w405]
      frame False {
      }
      frame True {
        w406 = FALSE
        n179 = shared-variable "roboRIO-1256-FRC\\Shared Variable.lvlib\\sendNewPic"(w407) -> ()  [unwired: 1 in, 1 out]
        n180 = xnode "Read/Write Control"("FPGA VI Reference In"=w405, "StartOfImage"=w407) -> ("FPGA VI Reference Out"=w408:refnum<k20>)  [unwired: 1 in, 1 out]
        n181 = xnode "Read/Write Control"("FPGA VI Reference In"=w408, "Ready For Output"=w407) -> ()  [unwired: 1 in, 2 out]
        n182 = shared-variable "roboRIO-1256-FRC\\Shared Variable.lvlib\\EndRecGaussian1"(w406) -> ()  [unwired: 1 in, 1 out]
        n183 = shared-variable "roboRIO-1256-FRC\\Shared Variable.lvlib\\EndRecGaussian2"(w406) -> ()  [unwired: 1 in, 1 out]
      }
    }
    n184 = xnode "Read/Write Control"("FPGA VI Reference In"=w395, "error in"=w382, "outputExtreme2"=w396) -> ("error out"=→"error out":errorcluster)  [unwired: 1 out]
  }
